vi "Get Tunnel Position on Structure_Flat Sequence.vi"(7 "Tunnel Type":enum16{"Tunnel", "FlatSeqInner", "FlatSeqOuter"}(ring), 8 "error in":errorcluster, 10 "FlatSeqOutTun Refnum":refnum<vi>, 11 "FlatSeqInTun Refnum":refnum<vi>) -> (0 "error out":errorcluster, 1 "Class Name":string, 3 "Tunnel Position":enum16{"Left", "Top", "Right", "Bottom"}(ring))   [LabVIEW 2023]
uses:
  <userlib>/_OpenG.lib/array/array.llb/openg_array.lvlib
panel:
  out "Structure Bounds":T1
  out "Position":cluster{"Left":i32, "Top":i32}
  # "debug"
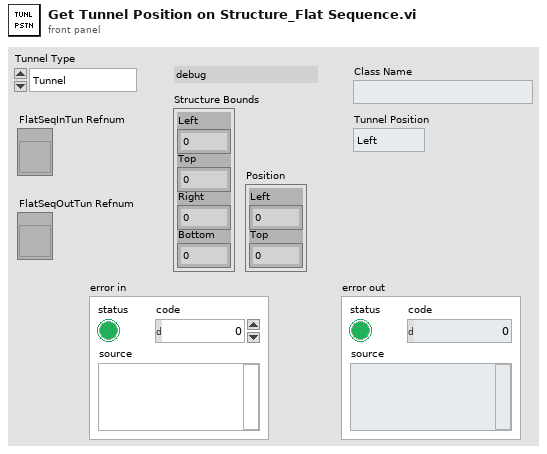
[diagram p1: front panel]
types:
  T1 = cluster{"Left":i16, "Top":i16, "Right":i16, "Bottom":i16}
  T2 = typedef "LVRectTypeDef.ctl" = cluster{"Left":i16, "Top":i16, "Right":i16, "Bottom":i16}
  T3 = typedef "LVPositionTypeDef.ctl" = cluster{"Left":i32, "Top":i32}
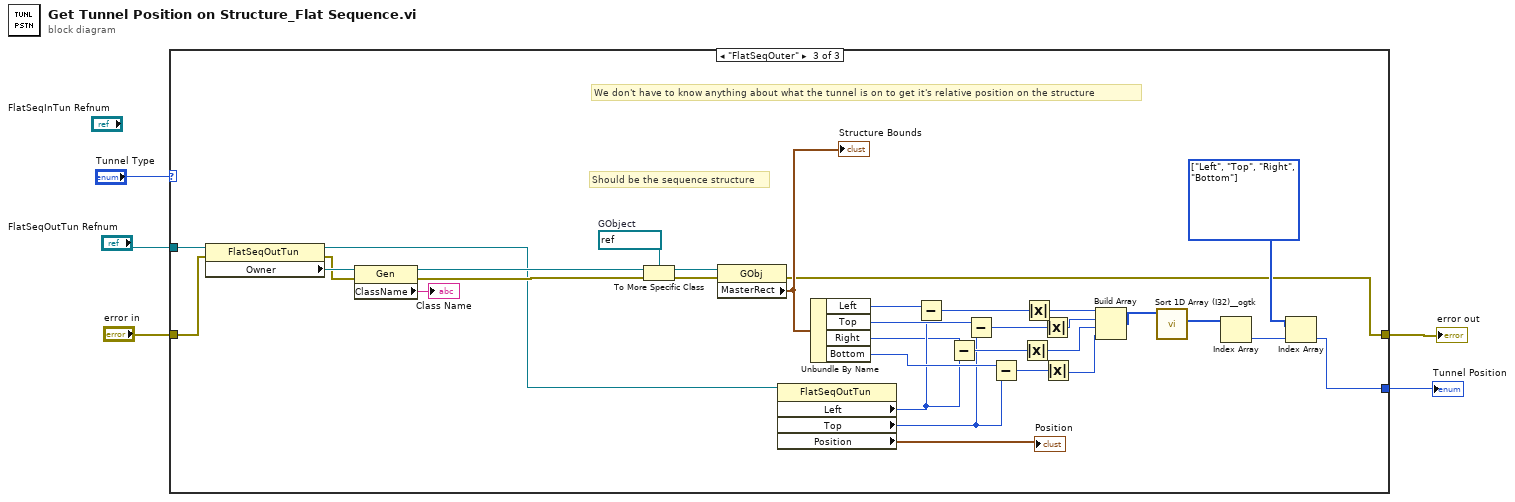
[diagram p0: block diagram]
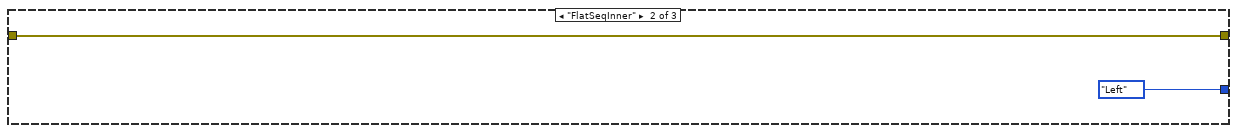
[diagram p3: hidden frame]
diagram:
  n1 = case shown="\"FlatSeqOuter\"" "Tunnel Type" {
    tunnel: [_ enum16{"Left", "Top", "Right", "Bottom"}."Left" ("Position") w40] -> w5
    tunnel: [w6 w7 w10] -> w4
    tunnel: "error in" -> [w6 w7 w35]
    tunnel: "FlatSeqOutTun Refnum" -> [_ _ w11]
    frame "Tunnel", Default {
    }
    frame "FlatSeqInner" {
    }
    frame "FlatSeqOuter" {
      w30 = enum16{"Left", "Top", "Right", "Bottom"}[] [enum."Left", enum."Top", enum."Right", enum."Bottom"] items=["Left", "Top", "Right", "Bottom"]
      w13 = refnum<vi> refnum  # GObject
      # "Should be the sequence structure"
      # "We don't have to know anything about what the tunnel is on to get it's relative position on the structure"
      n2 = property class="FlatSeqOutTun"(reference=w11, error in=w35) -> (reference out=w34:refnum<vi>, error out=w37:errorcluster, "Owner"=w39:refnum<vi>)
      n3 = property class="Gen"(reference=w39, error in=w37) -> (error out=w36:errorcluster, "ClassName"=→"Class Name":string)  [unwired: 1 out]
      n4 = To More Specific Class(target class=w13, reference=w39, error in=w36) -> (specific class reference=w14:refnum<vi>, error out=w12:errorcluster)
      n5 = property class="GObj"(reference=w14, error in=w12) -> (error out=w10:errorcluster, "MasterRect"=w33:T2)  [unwired: 1 out]
      "Structure Bounds" <- w33
      n6 = property class="FlatSeqOutTun"(reference=w34) -> ("Left"=w17:i32, "Top"=w19:i32, "Position"=→"Position":T3)  [unwired: 1 in, 2 out]
      n7 = Unbundle By Name(w33) -> ("Left"=w15:i16, "Top"=w18:i16, "Right"=w16:i16, "Bottom"=w20:i16)
      n8 = Subtract(x=w15, y=w17) -> (x-y=w21:i32)
      n9 = Subtract(x=w16, y=w17) -> (x-y=w23:i32)
      n10 = Subtract(x=w18, y=w19) -> (x-y=w22:i32)
      n11 = Subtract(x=w20, y=w19) -> (x-y=w24:i32)
      n12 = Absolute Value(x=w23) -> (abs(x)=w27:i32)
      n13 = Absolute Value(x=w21) -> (abs(x)=w25:i32)
      n14 = Absolute Value(x=w22) -> (abs(x)=w26:i32)
      n15 = Absolute Value(x=w24) -> (abs(x)=w28:i32)
      n16 = Build Array(w25, w26, w27, w28) -> (w29:i32[])
      n17 = call <userlib>:"Sort 1D Array (I32)__ogtk.vi"("Array in"=w29) -> ("Sorted Pointers"=w31:i32[])  [unwired: 9 in, 1 out]
      n18 = Index Array(array=w31) -> (element=w32:i32)  [unwired: 1 in]
      n19 = Index Array(array=w30, index=w32) -> (element=w40:enum16{"Left", "Top", "Right", "Bottom"})
    }
  }
  "Tunnel Position" <- w5
  "error out" <- w4
